vi "Validate DAQ model.vi"(8 "error in (no error)":errorcluster, 10 "Desired model":string="USB-6008", 11 "DAQ Module ID":i32) -> (0 "error out":errorcluster, 3 "Is model valid?":bool)   [LabVIEW 2020]
doc: "Validates whether the DAQ connected at the port is a desired DAQ model."
uses:
  Abeles-Brewster-Standa/NI_DAQ/Libraries/NI DAQ/NI DAQ.lvlib
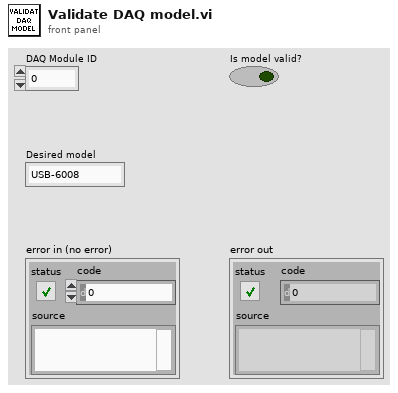
[diagram p1: front panel]
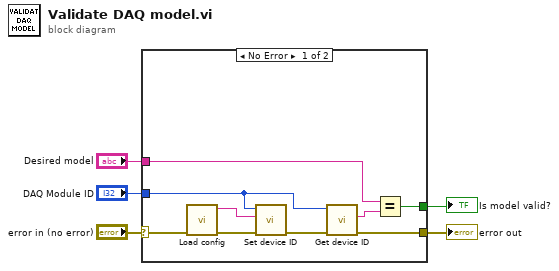
[diagram p0: block diagram]
diagram:
  n1 = case shown="No Error" "error in (no error)" {
    selector: "error in (no error)" -> [w7 w15]
    tunnel: [w13 _] -> w5
    tunnel: "DAQ Module ID" -> [w12 _]
    tunnel: [w11 w15] -> w3
    tunnel: "Desired model" -> [w6 _]
    frame No Error {
      n2 = call "Load config.vi"("error in (no error)"=w7) -> ("error out"=w8:errorcluster, "DAQ Port"=w9:tag)  [unwired: 9 in]
      n3 = call "Set device ID.vi"("error in"=w8, "Device ID"=w9, "Module ID"=w12) -> ("error out"=w10:errorcluster)  [unwired: 8 in]
      n4 = call "Get device ID.vi"("error in"=w10, "Module ID"=w12) -> ("error out"=w11:errorcluster, "Device ID"=w14:string)  [unwired: 7 in, 1 out]
      n5 = Equal?(x=w6, y=w14) -> (x = y?=w13:bool)
    }
    frame Error {
    }
  }
  "Is model valid?" <- w5
  "error out" <- w3
